vi "Fifo Read Bool Array.vi"(1 "latch":bool, 2 "index":i32, 3 "name":string) -> (0 "element":bool)   [LabVIEW 2012]
panel:
  out "empty?":bool
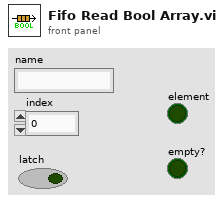
[diagram p1: front panel]
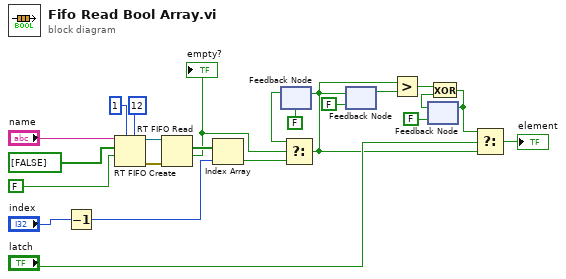
[diagram p0: block diagram]
diagram:
  n1 = Decrement(x="index") -> (x-1=w18:i32)
  n2 = RT FIFO Create(0:"name", 1:bool[] [FALSE], 2:FALSE ("create if not found? (T)"), 4:u32 1 ("size (10)"), 6:u32 12 ("elements in array (1)")) -> (8:w21:refnum<k33>, 11:w20:errorcluster)  [unwired: 3 in, 1 out]
  n3 = RT FIFO Read(0:w21, 3:w20) -> (9:w19:bool[], 10:w13:bool)  [unwired: 2 in, 3 out]
  "empty?" <- w13
  n4 = Index Array(array=w19, index=w18) -> (element=w12:bool)
  n5 = feedback #1(FALSE) -> (w11:bool)
  n6 = Select(t=w11, s=w13, f=w12) -> (s? t:f=w3:bool)
  n7 = feedback-in #1(w3) -> ()
  n8 = feedback-in #2(w3) -> ()
  n9 = feedback #2(FALSE) -> (w9:bool)
  n10 = Greater?(x=w3, y=w9) -> (0:w7:bool)
  n11 = feedback #3(FALSE) -> (w6:bool)
  n12 = Exclusive Or(1:w6, 2:w7) -> (0:w1:bool)
  n13 = feedback-in #3(w1) -> ()
  n14 = Select(t=w1, s="latch", f=w3) -> (s? t:f=→"element":bool)
